vi "while_loop.vi"() -> ()   [LabVIEW 2014]
panel:
  out "Loop #":i32
  in  "stop":bool
  out "LED1":bool
  out "LED2":bool
  in  "Inside Loop":bool
  in  "Outside Loop":bool
  in  "Knob":dbl(knob) scale=0.0..10.0
  out "Meter":dbl(knob) scale=0.0..10.0
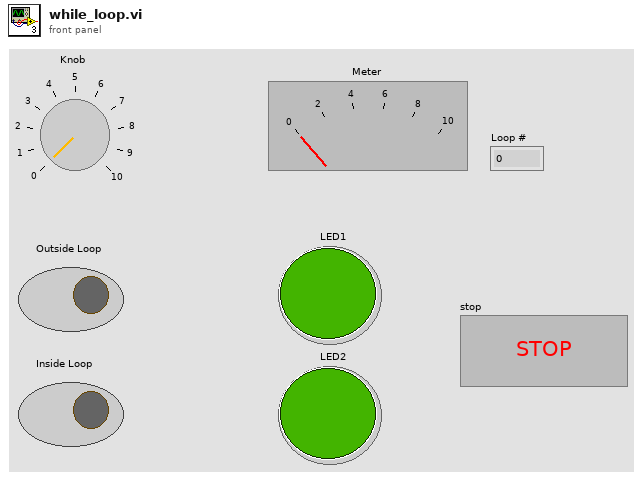
[diagram p1: front panel]
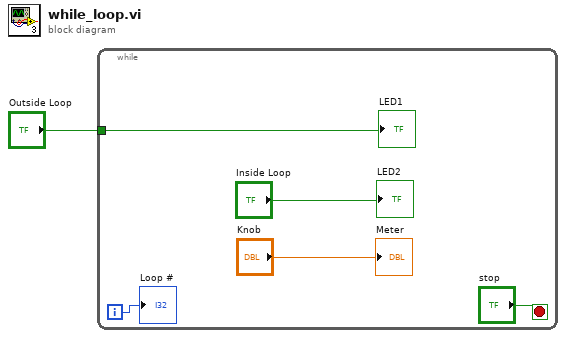
[diagram p0: block diagram]
diagram:
  n1 = while {
    tunnel: "Outside Loop" -> [w4]
    i -> [w2]
    stop <- "stop" stop-if-true
    "Meter" <- "Knob"
    "LED2" <- "Inside Loop"
    "LED1" <- w4
    "Loop #" <- w2
  }
